vi "Connect.vi"(8 "error in":errorcluster, 11 "LTB-1 in":refnum<class "LTB-1.lvclass">) -> (0 "error out":errorcluster, 3 "LTB-1 out":refnum<class "LTB-1.lvclass">)   [LabVIEW 2018, in "LTB-1.lvlib" / "LTB-1.lvclass"]
doc: "This is the parent method used to connect to the EXFO. The child class will override the function call and implement the appropriate methods as identified by the child class.\n\nAuthor: Ron Dexter\nCompany: Luminar\nModified: 5/20/2018"
uses:
  LTB-1.lvclass
  C:/AME Test Engineering/LabVIEW/PPLs/EXFO/Parent/EXFO.lvlibp/EXFO.lvclass
  PPLs/EXFO/Parent/EXFO.lvlibp/Methods/Read Resource.vi
  3150 Driver/3150.lvlib
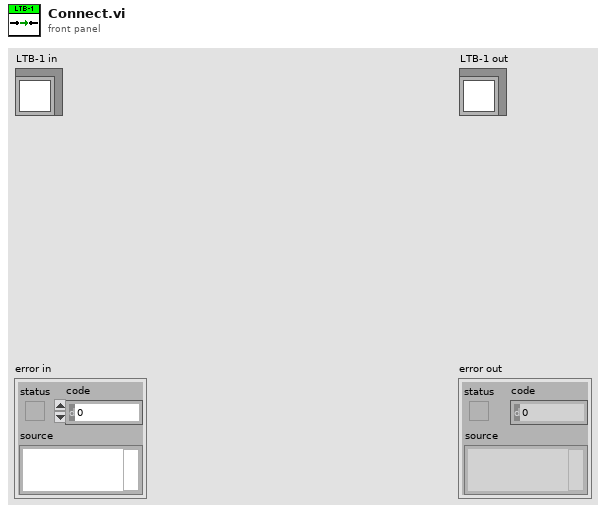
[diagram p1: front panel]
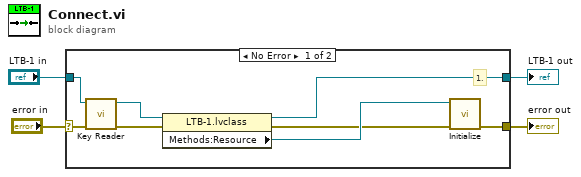
[diagram p0: block diagram]
diagram:
  n1 = case shown="No Error" "error in" {
    selector: "error in" -> [w11 w13]
    tunnel: "LTB-1 in" -> [w12 w14]
    tunnel: [w5 w14] -> w3
    tunnel: [w10 w13] -> w2
    frame No Error {
      # "1."
      n2 = call "Key Reader.vi"("error in"=w11, "LTB-1 in"=w12) -> ("error out"=w8:errorcluster, "LTB-1 out"=w9:refnum<class "LTB-1.lvclass">)  [unwired: 8 in]
      n3 = property class="LTB-1.lvclass"(reference=w9, error in=w8) -> (reference out=w5:refnum<class "LTB-1.lvclass">, error out=w6:errorcluster, "Methods:Resource"=w7:refnum<visa-resource-name>)
      n4 = call "Initialize.vi"("error in (no error)"=w6, "VISA resource name"=w7) -> ("error out"=w10:errorcluster)  [unwired: 8 in, 1 out]
    }
    frame Error {
    }
  }
  "error out" <- w2
  "LTB-1 out" <- w3
